vi "FinalBrain.vi"() -> ()   [LabVIEW 2012]
uses:
  <vilib>/imath/engines/lvmath/Plug In/_Char/NIMS_CH_character datatype.ctl
  <vilib>/Utility/inputDevices.llb/closeKeyboard.vi
  <vilib>/Utility/inputDevices.llb/keyboardAcquire.vi
  <vilib>/imath/engines/lvmath2/RunTimeEngine/ErrorHandling/NIMS_Finalize Error.vi
  <vilib>/imath/engines/lvmath2/RunTimeEngine/Managers/WorkSpace/UID Generator.vi
  <vilib>/imath/engines/lvmath2/RunTimeEngine/Managers/SymbolTable/Clear UID.vi
  <vilib>/imath/engines/lvmath2/RunTimeEngine/NodeEndStatement/NIMS_NodeEndStatement_Output.vi
  <instcachedir>/0/NIMS_NodeEndStatement_Output_53EC0D466D134D7ABD903AC30B43404B.lvgen/NIMS_NodeEndStatement_Output_53EC0D466D134D7ABD903AC30B43404B_010.vi
  <instcachedir>/0/NIMS_NodeEndStatement_Output_53EC0D466D134D7ABD903AC30B43404B.lvgen/NIMS_NodeEndStatement_Output_53EC0D466D134D7ABD903AC30B43404B_012.vi
  <vilib>/imath/engines/lvmath2/RunTimeEngine/RunTimeType/NIMS_RunTimeType_From StrictType (excl LVString).vi
  <instcachedir>/0/NIMS_RunTimeType_From StrictType (excl LVString)_AC52D965D0864706932D20A05968E122.lvgen/NIMS_RunTimeType_From StrictType (excl LVString)_AC52D965D0864706932D20A05968E122_000.vi
  <vilib>/imath/engines/lvmath2/RunTimeEngine/LocalVariableDefStatement/MC_LocalVariableDefStatement_Display.vi
  <vilib>/imath/engines/lvmath2/RunTimeEngine/RunTimeType/NIMS_RunTimeType_Set Source Original Bool.vi
  <vilib>/imath/engines/lvmath/Plug In/_Char/NIMS_CH_Character RV to String.vi
  <instcachedir>/0/NIMS_NodeEndStatement_Output_53EC0D466D134D7ABD903AC30B43404B.lvgen/NIMS_NodeEndStatement_Output_53EC0D466D134D7ABD903AC30B43404B_009.vi
  <instcachedir>/0/NIMS_RunTimeType_From StrictType (excl LVString)_AC52D965D0864706932D20A05968E122.lvgen/NIMS_RunTimeType_From StrictType (excl LVString)_AC52D965D0864706932D20A05968E122_001.vi
  <vilib>/imath/engines/lvmath2/RunTimeEngine/Managers/SymbolTable/NIMS_WorkSpace.lvlib
panel:
  out "Fully elapsed":bool
  out "Elapsed Time (s)":dbl
  out "String Received 3":string
  out "BS Timed Out":bool
  out "Base Station":string
  in  "error in (no error)":errorcluster
  in  "Tab Control":T1(tab)
  in  "Read Color":bool
  out "Bump Sensor 2":bool
  out "Distance 2, CM":dbl
  out "IR Volts Nav":dbl
  out "Red":dbl(knob) scale=0.0..50.0
  out "Green":dbl(knob) scale=0.0..50.0
  out "Blue":dbl(knob) scale=0.0..50.0
  out "Color Chosen":u32(colorbox)
  out "Bump Sensor 1":bool
  out "IR Volts Align":dbl
  out "Distance 1, CM":dbl
  in  "stop":bool
  out "Left Arm":i32
  out "Right Arm":i32
  in  "Arm":i32(slide)=1500 scale=500.0..2500.0
  out "Port\nMotor":i32
  out "Starboard\nMotor":i32
  out "Port Speed":i32(knob) scale=1000.0..2000.0
  out "Starboard Speed":i32(knob) scale=1000.0..2000.0
  out "Speed Balance":i32(knob) scale=-600.0..600.0
  in  "Numeric":i32=500
  in  "Arm Override":bool
  in  "Extend":bool
  in  "Initiate Mission":bool
  out "Angle to Target":i32
  out "Distance to Target":i32
  out "Bump 2":bool
  out "Bump  1":bool
  out "Current Target":i32
  out "Obstacle Detected":bool
  out "Primitive Engaged":string
  out "Desired Heading":i32
  out "Target Y":i32
  out "Target X":i32
  out "Current Y":i32
  out "Current X":i32
  out "Current Heading":i32
  out "Target Locations":i32[][](array[numeric])
  out "X Array":dbl[](array[numeric])
  out "Y Array":dbl[](array[numeric])
  in  "Step Size":i32=5
  in  "PC Status":i32=1
  out "String Received":string
  out "return count":u32
  out "bytes written":u32
  out "Blinky":bool
  in  "String":string="$CS1500P1500R1500L1500P1500H   1\n"
  in  "FULLSTOP":bool
  in  "VISA resource name":refnum<visa-resource-name>="COM7"
  # "ROBOT CONTROL VI\nSoftware Phase for Autonomy\n\nVPreston\n4/14/2014"
  # "Thought:\n- Need to calibrate the accelerometer each time, which means that the first step will need to be \nSpinning in place at a set location (likely the landing zone)\n- Is this worth it?  If not, a simple heading can be developed based upon movement from the \ncamera, though this is likely to be glitchy and less reliable....\n\n- Calculate heading with accelerometer in the hindbrain, pass this up to PC\nOR\n- Calculate heading from base station in PC"
  # "Use this tab to make sure your sensors are happy and working properly."
  # "Motor Control"
  # "Direction of thrust"
  # "Purple Target - 80, 230\nYellow Target - \nRed Target - 37, 78 \nGreen Target - 258, 43 \nBlue Target - 492, 63"
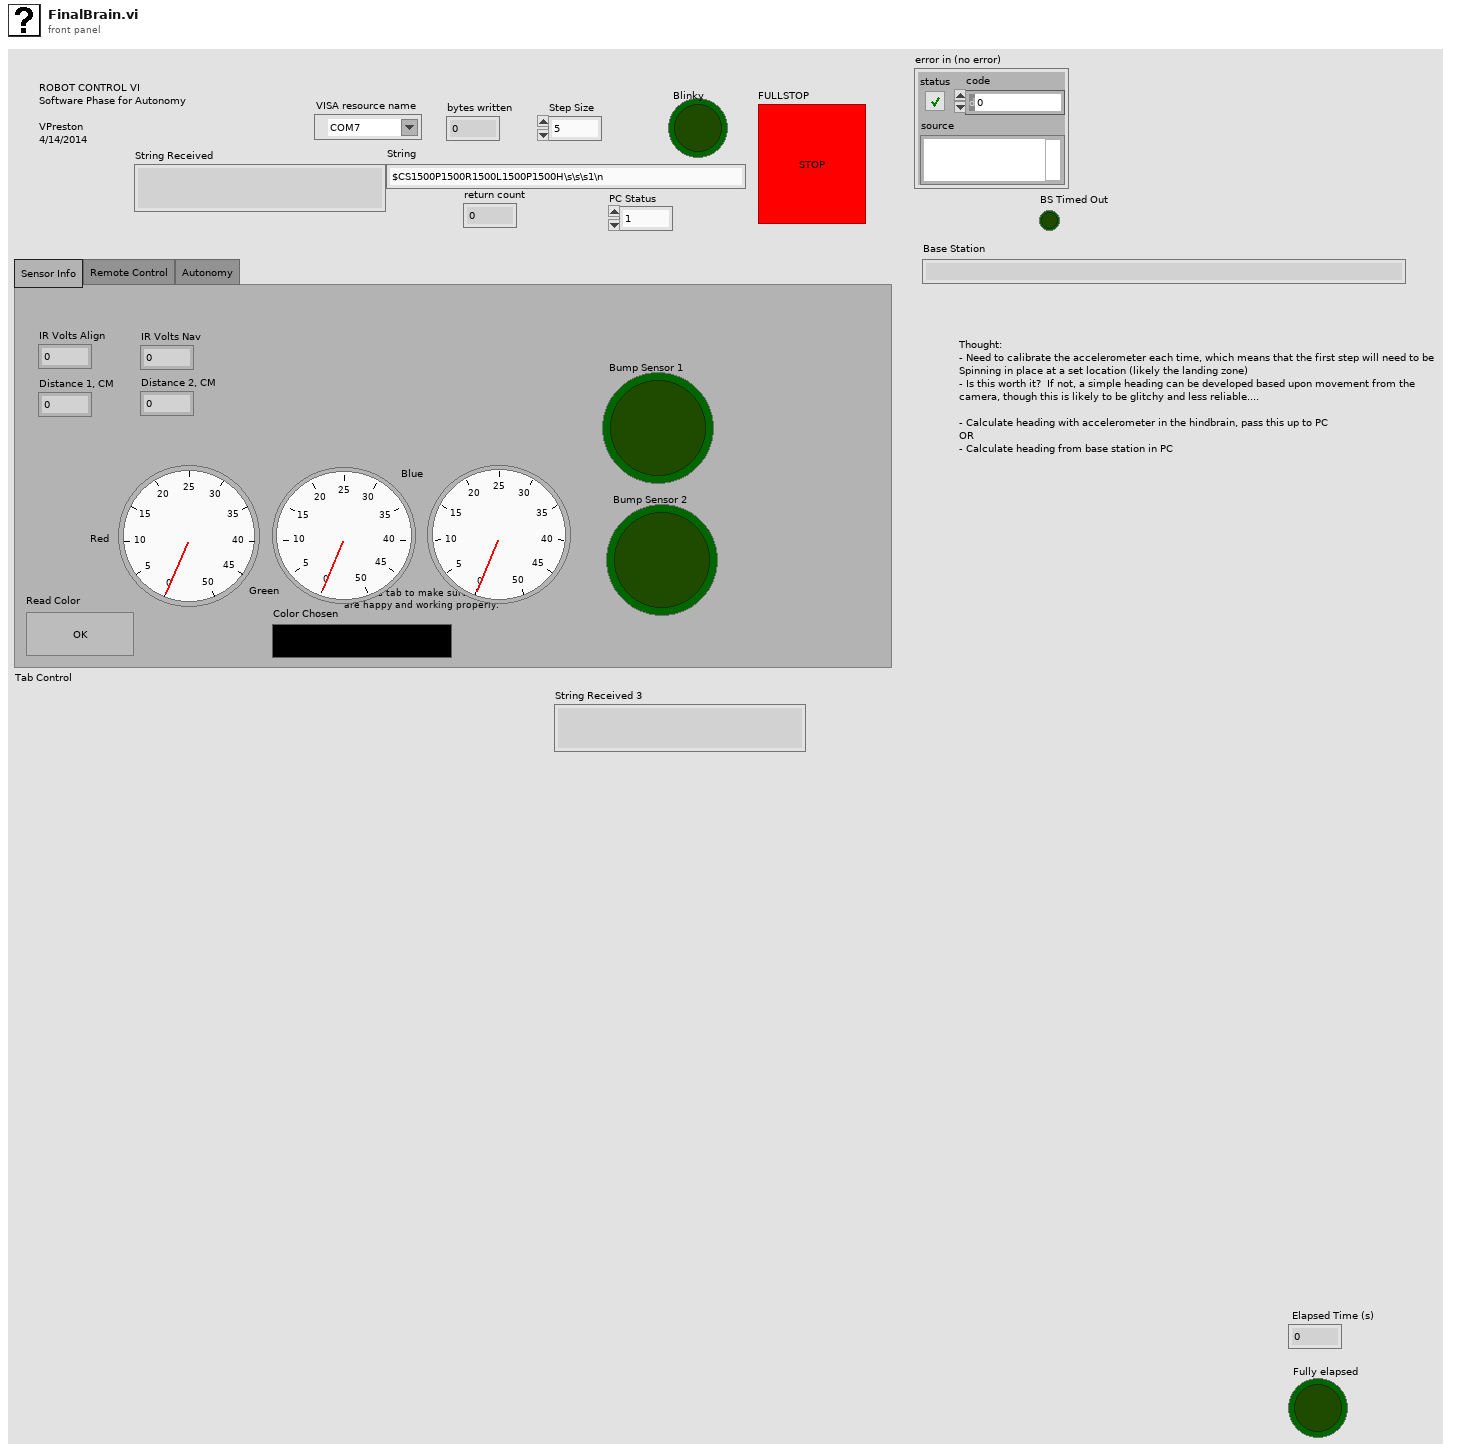
[diagram p1: front panel]
types:
  T1 = enum32{"Sensor Info", "Remote Control", "Autonomy"}
  T2 = enum16{"0", "1", "2", "3", "4", "5", "6", "7", "8", "9", "A", "B", "C", "D", "E", "F", "G", "H", "I", "J", "K", "L", "M", "N", "O", "P", "Q", "R", "S", "T", "U", "V", "W", "X", "Y", "Z", "F1", "F2", "F3", "F4", "F5", "F6", "F7", "F8", "F9", "F10", "F11", "F12", "F13", "F14", "F15", "ADD", "BACK", "BACKSLASH", "CAPITAL", "COMMA", "DECIMAL", "DELETE", "DIVIDE", "DOWN", "END", "EQUALS", "ESCAPE", "GRAVE (`)", "HOME", "INSERT", "LBRACKET", "LCONTROL", "LEFT", "L ALT", "LSHIFT", "LWIN", "MINUS", "MULTIPLY", "NEXT", "NUMLOCK", "NUMPAD_0", "NUMPAD_1", "NUMPAD_2", "NUMPAD_3", "NUMPAD_4", "NUMPAD_5", "NUMPAD_6", "NUMPAD_7", "NUMPAD_8", "NUMPAD_9", "PAUSE", "PERIOD", "PRIOR (PG UP)", "RBRACKET", "RCONTROL", "RETURN", "RIGHT", "R ALT", "RSHIFT", "RWIN", "SCROLL", "SEMICOLON", "SLASH", "SPACE", "SUBTRACT", "TAB", "UP", "ENTER (num pad)", "' (quote)"}[]
  T3 = enum16{"0", "1", "2", "3", "4", "5", "6", "7", "8", "9", "A", "B", "C", "D", "E", "F", "G", "H", "I", "J", "K", "L", "M", "N", "O", "P", "Q", "R", "S", "T", "U", "V", "W", "X", "Y", "Z", "F1", "F2", "F3", "F4", "F5", "F6", "F7", "F8", "F9", "F10", "F11", "F12", "F13", "F14", "F15", "ADD", "BACK", "BACKSLASH", "CAPITAL", "COMMA", "DECIMAL", "DELETE", "DIVIDE", "DOWN", "END", "EQUALS", "ESCAPE", "GRAVE (`)", "HOME", "INSERT", "LBRACKET", "LCONTROL", "LEFT", "L ALT", "LSHIFT", "LWIN", "MINUS", "MULTIPLY", "NEXT", "NUMLOCK", "NUMPAD_0", "NUMPAD_1", "NUMPAD_2", "NUMPAD_3", "NUMPAD_4", "NUMPAD_5", "NUMPAD_6", "NUMPAD_7", "NUMPAD_8", "NUMPAD_9", "PAUSE", "PERIOD", "PRIOR (PG UP)", "RBRACKET", "RCONTROL", "RETURN", "RIGHT", "R ALT", "RSHIFT", "RWIN", "SCROLL", "SEMICOLON", "SLASH", "SPACE", "SUBTRACT", "TAB", "UP", "ENTER (num pad)", "' (quote)"}
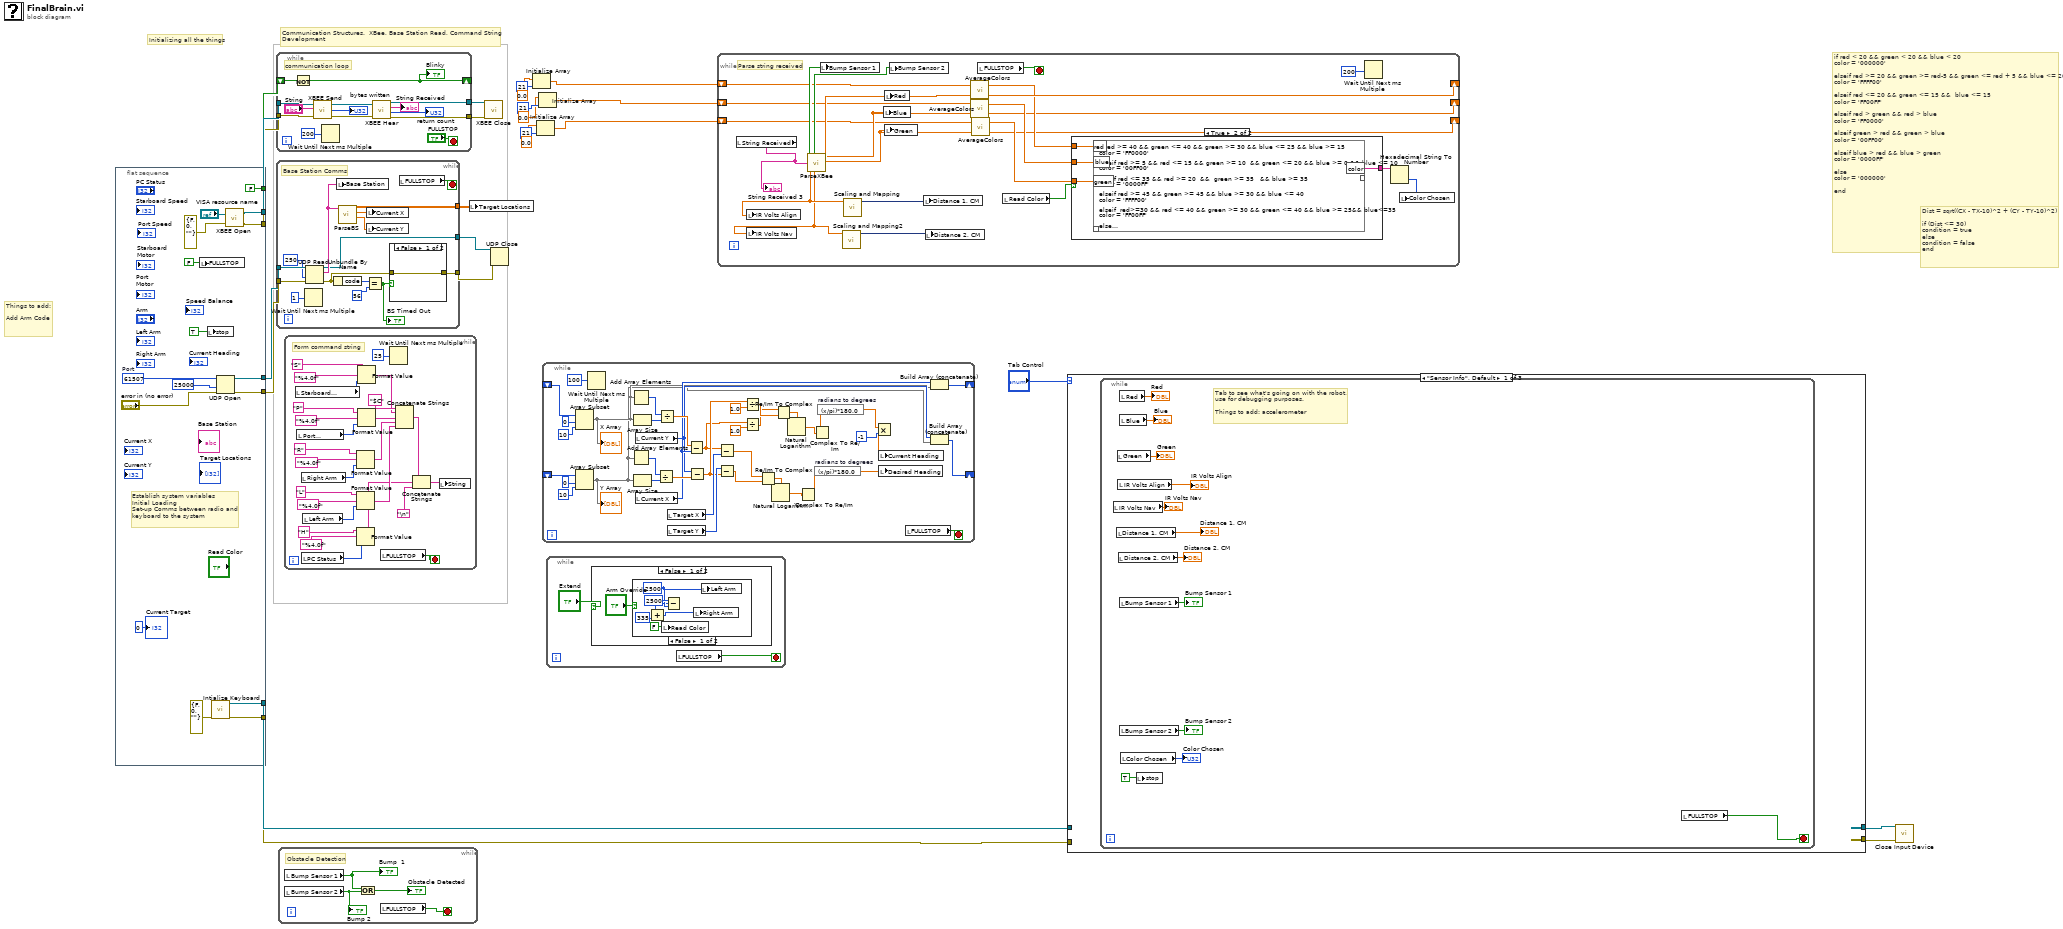
[diagram p0: block diagram]
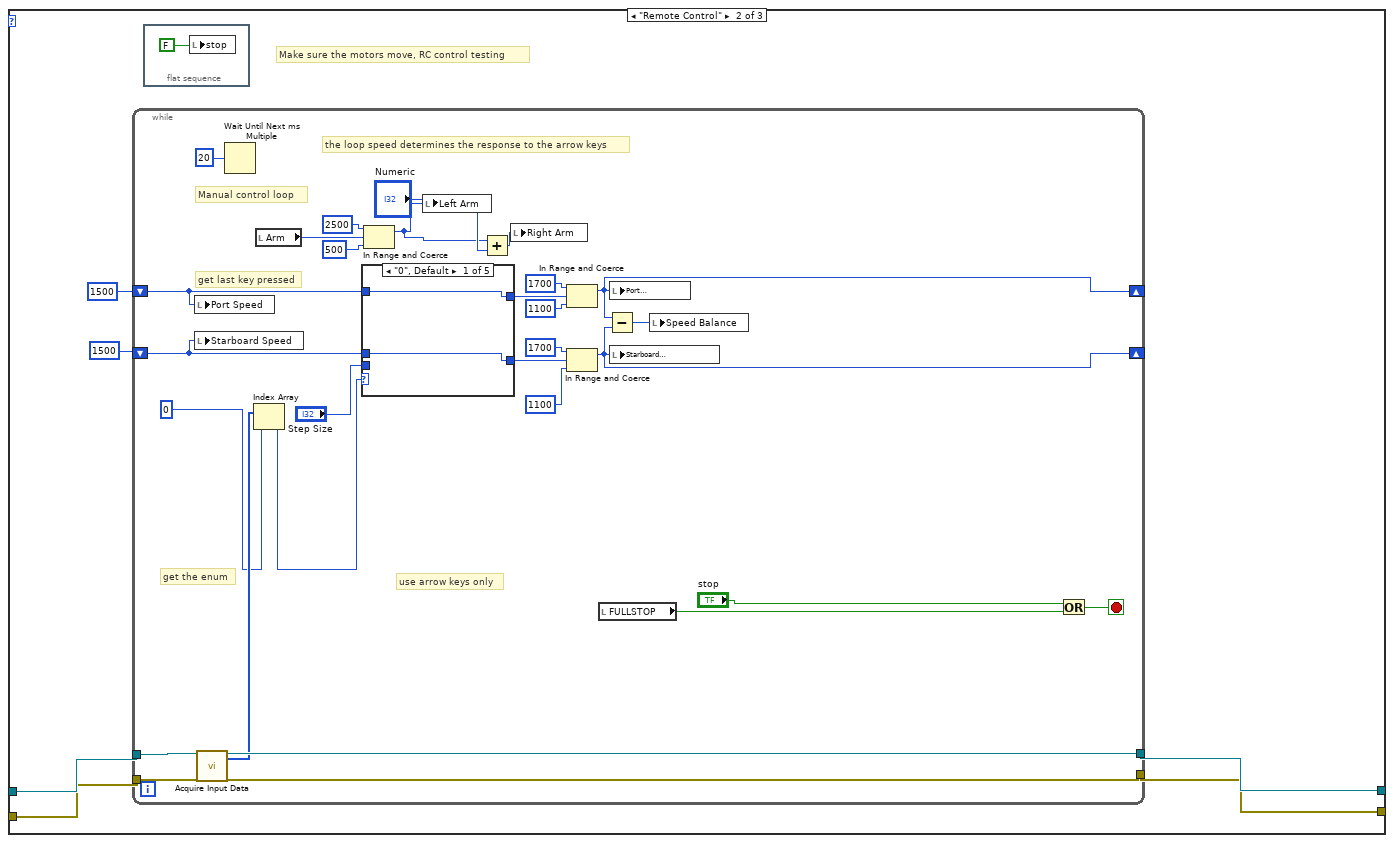
[diagram p2: hidden frame]
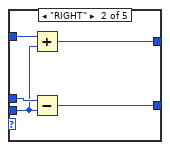
[diagram p3: hidden frame]
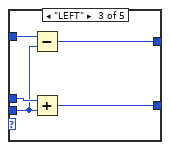
[diagram p4: hidden frame]
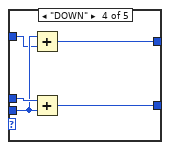
[diagram p5: hidden frame]
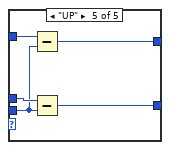
[diagram p6: hidden frame]
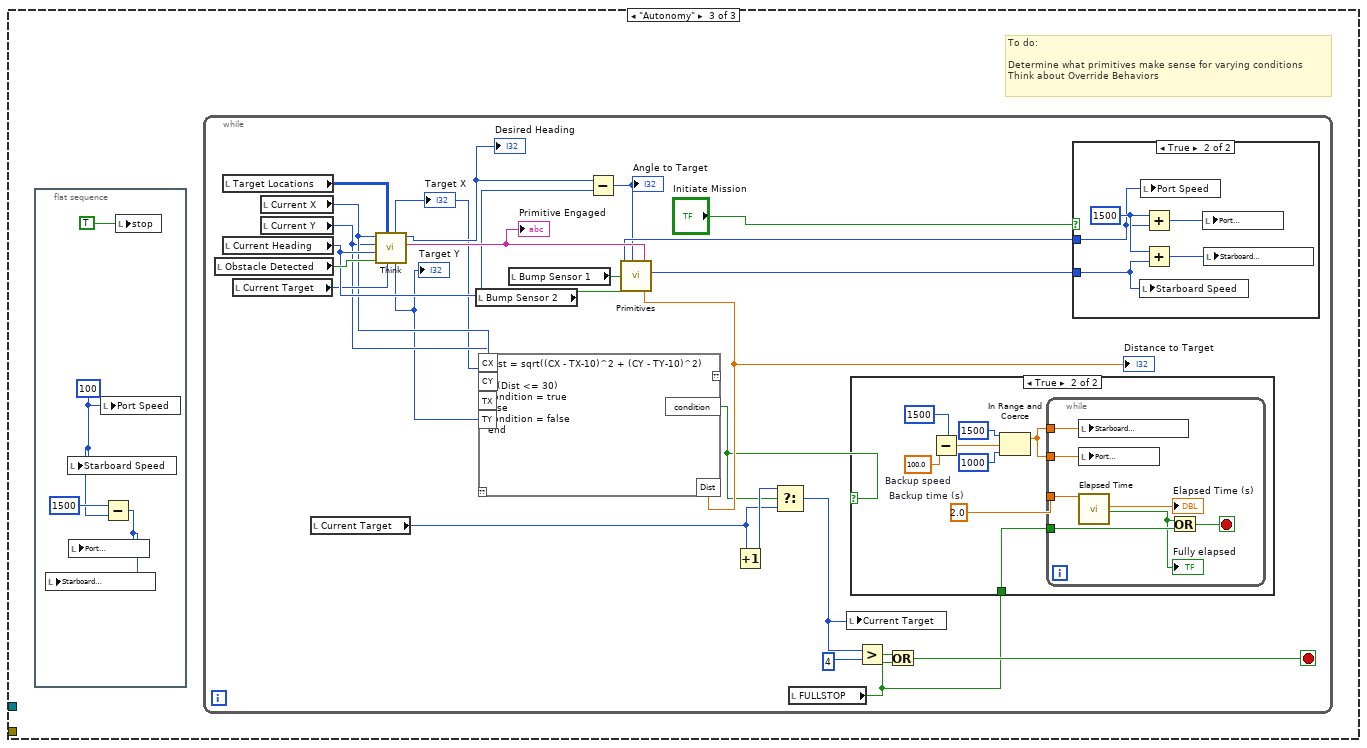
[diagram p7: hidden frame]
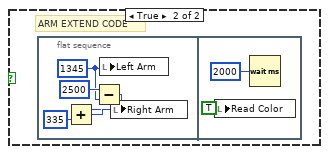
[diagram p11: hidden frame]
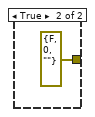
[diagram p12: hidden frame]
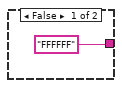
[diagram p13: hidden frame]
diagram:
  # "Dist = sqrt((CX - TX-10)^2 + (CY - TY-10)^2)\n\nif (Dist <= 30)\ncondition = true\nelse\ncondition = false\nend"
  # "if red < 20 && green < 20 && blue < 20\ncolor = '000000'\n\nelseif red >= 20 && green >= red-5 && green <= red + 5 && blue <= 20\ncolor = 'FFFF00'\n\nelseif red <= 20 && green <= 15 &&  blue <= 15\ncolor = 'FF00FF'\n\nelseif red > green && red > blue\ncolor = 'FF0000'\n\nelseif green > red && green > blue\ncolor = '00FF00'\n\nelseif blue > red && blue > green\ncolor = '0000FF' \n\nelse\ncolor = '000000'\n\nend"
  # "Initializing all the things"
  # "Communication Structures.  XBee, Base Station Read, Command String Development"
  # "Things to add: \n\nAdd Arm Code"
  n1 = flat-sequence {
    tunnel: [w40] -> w24
    tunnel: [w28] -> w23
    tunnel: [FALSE] -> w20
    tunnel: [w35] -> w19
    tunnel: [w34] -> w18
    tunnel: [w27] -> w12
    tunnel: [w29] -> w15
    frame #0 {
      w31 = u16 61507  # Port
      # "Establish system variables\nInitial Loading\nSet-up Comms between radio and\nkeyboard to the system"
      n2 = local write "FULLSTOP"(FALSE) -> ()
      n3 = local write "stop"(TRUE) -> ()
      n4 = call <vilib>:"Intialize Keyboard.vi"("error in (no error)"=errorcluster {"status"=FALSE, "code"=0, "source"=""}) -> ("error out"=w34:errorcluster, "device ID"=w35:refnum<k1>)  [unwired: 9 in]
      n5 = UDP Open(8:"error in (no error)", 9:25000 ("timeout ms (25000)"), 11:w31) -> (port=w27:refnum<k16>, 0:w29:errorcluster)  [unwired: 2 in, 1 out]
      n6 = call "XBEE Open.vi"("error in"=errorcluster {"status"=FALSE, "code"=0, "source"=""}, "VISA resource name"="VISA resource name") -> ("error out"=w28:errorcluster, "VISA resource name out"=w40:refnum<visa-resource-name>)
      "Current Target" <- 0
    }
  }
  n7 = while {
    tunnel: w24 -> [w53]
    tunnel: w23 -> [w52]
    tunnel: [w47] -> w22
    tunnel: [w46] -> w21
    shift-right: [w50] -> _
    shift-left: w20 -> [w51]
    stop <- "FULLSTOP" stop-if-true
    # "communication loop"
    n8 = Not(x=w51) -> (.not. x?=w50:bool)
    "Blinky" <- w50
    n9 = call "XBEE Send.vi"("error in (no error)"=w52, "String"="String", "VISA resource name"=w53) -> ("error out"=w43:errorcluster, "return count"=→"bytes written":u32, "VISA resource name out"=w44:refnum<visa-resource-name>)
    n10 = Wait Until Next ms Multiple(millisecond multiple=u32 200) -> ()  [unwired: 1 out]
    n11 = call "XBEE Hear.vi"("VISA resource name"=w44, "error in (no error)"=w43) -> ("VISA resource name out"=w47:refnum<visa-resource-name>, "String Received"=→"String Received":string, "return count"=→"return count":u32, "error out"=w46:errorcluster)
  }
  n12 = while {
    tunnel: w12 -> [w69]
    tunnel: w15 -> [w68]
    tunnel: [w57] -> w14
    tunnel: [w56] -> w13
    tunnel: [w55] -> w1
    stop <- w61 stop-if-true
    # "Base Station Comms"
    n13 = Wait Until Next ms Multiple(millisecond multiple=u32 1) -> ()  [unwired: 1 out]
    n14 = UDP Read(connection ID=w69, timeout ms (25000)=250, 8:w68) -> (data out=w60:string, error out=w64:errorcluster, 3:w57:refnum<k16>)  [unwired: 1 in, 2 out]
    n15 = Unbundle By Name(w64) -> ("code"=w63:i32)
    n16 = local write "Base Station"(w60) -> ()
    n17 = call "ParseBS.vi"("BS String"=w60) -> ("Y Pos"=w58:dbl, "X Pos"=w59:dbl, "Targets!"=w55:dbl[][])  [unwired: 7 in]
    n18 = Equal?(x=w63, y=56) -> (x = y?=w62:bool)
    "BS Timed Out" <- w62
    n19 = local write "Current X"(w59) -> ()
    n20 = local write "Current Y"(w58) -> ()
    n21 = case shown="False" w62 {
      tunnel: [w70 errorcluster {"status"=FALSE, "code"=0, "source"=""} ("error out")] -> w56
      tunnel: w64 -> [w70 _]
      frame False {
      }
      frame True {
      }
    }
    n22 = local read "FULLSTOP"() -> (w61:bool)
  }
  n23 = while {
    stop <- w75 stop-if-true
    # "Obstacle Detection"
    n24 = local read "Bump Sensor 1"() -> (w74:bool)
    "Bump  1" <- w74
    n25 = local read "Bump Sensor 2"() -> (w73:bool)
    "Bump 2" <- w73
    n26 = Or(x=w74, y=w73) -> (x .or. y?=→"Obstacle Detected":bool)
    n27 = local read "FULLSTOP"() -> (w75:bool)
  }
  n28 = while {
    stop <- w101 stop-if-true
    # "Form command string"
    n29 = local read "Starboard\nMotor"() -> (w98:i32)
    n30 = local read "Port\nMotor"() -> (w95:i32)
    n31 = local read "Right Arm"() -> (w89:i32)
    n32 = local read "PC Status"() -> (w80:i32)
    n33 = local read "Left Arm"() -> (w86:i32)
    n34 = Format Value(string ("")="R", format string="%4.0f", value (0)=w89) -> (output string=w85:string)
    n35 = Format Value(string ("")="H", format string="%4.0f", value (0)=w80) -> (output string=w77:string)
    n36 = Format Value(string ("")="L", format string="%4.0f", value (0)=w86) -> (output string=w84:string)
    n37 = Format Value(string ("")="S", format string="%4.0f", value (0)=w98) -> (output string=w93:string)
    n38 = Format Value(string ("")="P", format string="%4.0f", value (0)=w95) -> (output string=w92:string)
    n39 = local read "FULLSTOP"() -> (w101:bool)
    n40 = Wait Until Next ms Multiple(millisecond multiple=u32 25) -> ()  [unwired: 1 out]
    n41 = Concatenate Strings("$C", w93, w92, w85, w84) -> (w79:string)
    n42 = Concatenate Strings(w79, w77, "\n") -> (w83:string)
    n43 = local write "String"(w83) -> ()
  }
  n44 = local write "Target Locations"(w1) -> ()
  n45 = call "XBEE Close.vi"("error in (no error)"=w21, "VISA resource name"=w22) -> ()
  n46 = UDP Close(connection ID=w14, 8:w13) -> ()  [unwired: 2 out]
  n47 = Initialize Array(0.0 ("element"), 21 ("dimension size")) -> (w11:dbl[])
  n48 = Initialize Array(0.0 ("element"), 21 ("dimension size")) -> (w3:dbl[])
  n49 = Initialize Array(0.0 ("element"), 21 ("dimension size")) -> (w4:dbl[])
  n50 = while {
    shift-right: [w121] -> _
    shift-left: _ -> [w141]
    shift-right: [w118] -> _
    shift-left: _ -> [w135]
    stop <- w134 stop-if-true
    n51 = Array Subset(array=w141, index=0, length=10) -> (w117:i32[])
    "X Array" <- w117
    n52 = Array Subset(array=w135, index=0, length=10) -> (w116:i32[])
    "Y Array" <- w116
    n53 = Wait Until Next ms Multiple(millisecond multiple=100) -> ()  [unwired: 1 out]
    n54 = Add Array Elements(numeric array=w117) -> (sum=w132:i32)
    n55 = Add Array Elements(numeric array=w116) -> (sum=w130:i32)
    n56 = Array Size(array=w117) -> (size(s)=w131:i32)
    n57 = Array Size(array=w116) -> (size(s)=w129:i32)
    n58 = local read "Current Y"() -> (w119:i32)
    n59 = local read "Current X"() -> (w120:i32)
    n60 = Divide(x=w130, y=w129) -> (x/y=w124:dbl)
    n61 = Divide(x=w132, y=w131) -> (x/y=w122:dbl)
    n62 = local read "Target X"() -> (w126:i32)
    n63 = local read "Target Y"() -> (w125:i32)
    n64 = Subtract(x=w122, y=w120) -> (x-y=w115:dbl)
    n65 = Subtract(x=w119, y=w124) -> (x-y=w123:dbl)
    n66 = Subtract(x=w115, y=w126) -> (x-y=w104:dbl)
    n67 = Subtract(x=w125, y=w123) -> (x-y=w105:dbl)
    n68 = Divide(x=w123, y=1.0) -> (x/y=w111:dbl)
    n69 = Divide(x=w115, y=1.0) -> (x/y=w110:dbl)
    n70 = Re/Im To Complex(1:w105, 2:w104) -> (0:w106:cdb)
    n71 = Natural Logarithm(1:w106) -> (0:w103:cdb)
    n72 = Re/Im To Complex(1:w111, 2:w110) -> (0:w109:cdb)
    n73 = Natural Logarithm(1:w109) -> (0:w108:cdb)
    n74 = Complex To Re/Im(x + iy=w103) -> (y=w102:dbl)  [unwired: 1 out]
    n75 = Complex To Re/Im(x + iy=w108) -> (y=w107:dbl)  [unwired: 1 out]
    n76 = expression code="(x/pi)*180.0" "radians to degrees"(w102) -> (w133:dbl)
    n77 = expression code="(x/pi)*180.0" "radians to degrees"(w107) -> (w113:dbl)
    n78 = Multiply(x=w113, y=-1) -> (x*y=w112:dbl)
    n79 = local write "Current Heading"(w112) -> ()
    n80 = local write "Desired Heading"(w133) -> ()
    n81 = local read "FULLSTOP"() -> (w134:bool)
    n82 = Build Array (concatenate)(w120, w117) -> (w121:i32[])
    n83 = Build Array (concatenate)(w119, w116) -> (w118:i32[])
  }
  n84 = while {
    stop <- w143 stop-if-true
    n85 = case shown="False" "Extend" {
      frame False {
        n86 = case shown="False" "Arm Override" {
          frame False {
            w148 = 2500 ("Left Arm")
            n87 = local write "Read Color"(FALSE ("Read Color")) -> ()
            n88 = Subtract(x=2500, y=w148) -> (x-y=w147:i32)
            n89 = Add(x=w147, y=335) -> (x+y=w146:i32)
            n90 = local write "Right Arm"(w146) -> ()
            n91 = local write "Left Arm"(w148) -> ()
          }
          frame True {
          }
        }
      }
      frame True {
        # "ARM EXTEND CODE"
        n92 = flat-sequence {
          frame #0 {
            w152 = 1345 ("Left Arm")
            n93 = Subtract(x=2500, y=w152) -> (x-y=w153:i32)
            n94 = Add(x=w153, y=335) -> (x+y=w154:i32)
            n95 = local write "Left Arm"(w152) -> ()
            n96 = local write "Right Arm"(w154) -> ()
          }
          frame #1 {
            n97 = local write "Read Color"(TRUE ("Read Color")) -> ()
            n98 = Wait (ms)(milliseconds to wait=u32 2000) -> ()  [unwired: 1 out]
          }
        }
      }
    }
    n99 = local read "FULLSTOP"() -> (w143:bool)
  }
  n100 = while {
    shift-right: [w171] -> _
    shift-left: w11 -> [w172]
    shift-right: [w163] -> _
    shift-left: w4 -> [w164]
    shift-right: [w161] -> _
    shift-left: w3 -> [w162]
    stop <- w165 stop-if-true
    # "Parse string received"
    n101 = local read "String Received"() -> (w159:string)
    "String Received 3" <- w159
    n102 = call "ParseXBee.vi"("XBee String"=w159) -> ("Bump 1"=w177:bool, "Bump 2"=w176:bool, "IR Align"=w175:dbl, "IR Nav"=w174:dbl, "Red"=w173:dbl, "Blue"=w169:dbl, "Green"=w167:dbl)  [unwired: 3 in]
    n103 = local write "IR Volts Align"(w175) -> ()
    n104 = local write "IR Volts Nav"(w174) -> ()
    n105 = local write "Bump Sensor 1"(w177) -> ()
    n106 = call "Scaling and Mapping2"("Signals"=w174) -> ("Scaled Signals"=w178:dynamicdata)  [unwired: 9 in, 1 out]
    n107 = call "Scaling and Mapping"("Signals"=w175) -> ("Scaled Signals"=w179:dynamicdata)  [unwired: 9 in, 1 out]
    n108 = local write "Blue"(w169) -> ()
    n109 = local write "Red"(w173) -> ()
    n110 = local write "Green"(w167) -> ()
    n111 = local write "Bump Sensor 2"(w176) -> ()
    n112 = local write "Distance 1, CM"(w179) -> ()
    n113 = local write "Distance 2, CM"(w178) -> ()
    n114 = call "AverageColors.vi"("ColorData"=w173, "CurrentArray"=w172) -> ("UpdatedArray"=w171:dbl[], "Average"=w170:dbl)
    n115 = call "AverageColors.vi"("ColorData"=w169, "CurrentArray"=w164) -> ("UpdatedArray"=w163:dbl[], "Average"=w168:dbl)
    n116 = call "AverageColors.vi"("ColorData"=w167, "CurrentArray"=w162) -> ("UpdatedArray"=w161:dbl[], "Average"=w166:dbl)
    n117 = local read "FULLSTOP"() -> (w165:bool)
    n118 = local read "Read Color"() -> (w160:bool)
    n119 = case shown="True" w160 {
      tunnel: ["FFFFFF" w186] -> w181
      tunnel: w170 -> [_ w185]
      tunnel: w168 -> [_ w184]
      tunnel: w166 -> [_ w183]
      frame False {
      }
      frame True {
        n120 = mathscript code="if red >= 40 && green <= 40 && green >= 30 && blue <= 25 && blue >= 15\ncolor = 'FF0000'\n\nelseif red >= 5 && red <= 15 && green >= 10  && green <= 20 && blue >= 0 && blue <= 10\ncolor = '00FF00'\n\nelseif red <= 35 && red >= 20  &&  green >= 35   && blue >= 35 \ncolor = '0000FF'\n\nelseif red >= 45 && green >= 45 && blue >= 30 && blue <= 40\ncolor = 'FFFF00'\n\nelseif  red>=30 && red <= 40 && green >= 30 && green <= 40 && blue >= 25&& blue<=35\ncolor = 'FF00FF'\n\nelse\ncolor = '000000'\n\nend"("red"=w185, "blue"=w184, "green"=w183) -> ("color"=w186:string)  [unwired: 1 in, 1 out]
      }
    }
    n121 = Wait Until Next ms Multiple(millisecond multiple=200) -> ()  [unwired: 1 out]
    n122 = Hexadecimal String To Number(string=w181) -> (number=w180:u32)  [unwired: 2 in, 1 out]
    n123 = local write "Color Chosen"(w180) -> ()
  }
  n124 = case shown="\"Sensor Info\", Default" "Tab Control" {
    tunnel: w19 -> [_ w540 _]
    tunnel: w18 -> [_ w539 _]
    tunnel: [_ w536 _] -> w17
    tunnel: [_ w535 _] -> w16
    frame "Sensor Info", Default {
      n125 = while {
        stop <- w523 stop-if-true
        # "Tab to see what's going on with the robot, \nuse for debugging purposes.  \n\nThings to add: accelerometer"
        n126 = local read "IR Volts Nav"() -> (→"IR Volts Nav":dbl)
        n127 = local read "Distance 1, CM"() -> (→"Distance 1, CM":dbl)
        n128 = local read "Green"() -> (→"Green":dbl)
        n129 = local read "IR Volts Align"() -> (→"IR Volts Align":dbl)
        n130 = local read "Distance 2, CM"() -> (→"Distance 2, CM":dbl)
        n131 = local read "Bump Sensor 1"() -> (→"Bump Sensor 1":bool)
        n132 = local read "Bump Sensor 2"() -> (→"Bump Sensor 2":bool)
        n133 = local read "Red"() -> (→"Red":dbl)
        n134 = local read "Blue"() -> (→"Blue":dbl)
        n135 = local read "Color Chosen"() -> (→"Color Chosen":u32)
        n136 = local write "stop"(TRUE) -> ()
        n137 = local read "FULLSTOP"() -> (w523:bool)
      }
    }
    frame "Remote Control" {
      # "Make sure the motors move, RC control testing"
      n138 = while {
        tunnel: [w570] -> w535
        tunnel: [w569] -> w536
        shift-right: [w553] -> _
        shift-left: 1500 -> [w555]
        shift-right: [w552] -> _
        shift-left: 1500 -> [w554]
        tunnel: w540 -> [w546]
        tunnel: w539 -> [w545]
        stop <- w547 stop-if-true
        # "use arrow keys only"
        # "Manual control loop"
        # "get the enum"
        # "the loop speed determines the response to the arrow keys"
        # "get last key pressed"
        n139 = local write "Port Speed"(w554) -> ()
        n140 = local write "Starboard Speed"(w555) -> ()
        n141 = call-poly <vilib>:"Acquire Input Data.vi"("device ID"=w546, "error in (no error)"=w545) -> ("device ID"=w569:refnum<k1>, "keys pressed"=w568:T2, "error out"=w570:errorcluster)  [unwired: 15 in]
        n142 = Wait Until Next ms Multiple(millisecond multiple=u32 20) -> ()  [unwired: 1 out]
        n143 = Index Array(array=w568, index=0) -> (element=w566:T3)
        n144 = local read "Arm"() -> (w550:i32)
        n145 = case shown="\"0\", Default" w566 {
          tunnel: w555 -> [w572 w574 w579 w587 w592]
          tunnel: [w572 w575 w580 w586 w591] -> w564
          tunnel: w554 -> [w571 w577 w581 w584 w590]
          tunnel: [w571 w576 w582 w583 w588] -> w556
          tunnel: "Step Size" -> [_ w573 w578 w585 w589]
          frame "0", Default {
          }
          frame "RIGHT" {
            n146 = Add(x=w577, y=w573) -> (x+y=w576:i32)
            n147 = Subtract(x=w574, y=w573) -> (x-y=w575:i32)
          }
          frame "LEFT" {
            n148 = Subtract(x=w581, y=w578) -> (x-y=w582:i32)
            n149 = Add(x=w579, y=w578) -> (x+y=w580:i32)
          }
          frame "DOWN" {
            n150 = Add(x=w585, y=w584) -> (x+y=w583:i32)
            n151 = Add(x=w587, y=w585) -> (x+y=w586:i32)
          }
          frame "UP" {
            n152 = Subtract(x=w590, y=w589) -> (x-y=w588:i32)
            n153 = Subtract(x=w592, y=w589) -> (x-y=w591:i32)
          }
        }
        n154 = In Range and Coerce(upper limit=2500, x=w550, lower limit=500) -> (coerced(x)=w542:i32)  [unwired: 1 out]
        n155 = local write "Left Arm"(w542) -> ()
        n156 = Add(x=w542, y="Numeric") -> (x+y=w543:i32)
        n157 = local write "Right Arm"(w543) -> ()
        n158 = In Range and Coerce(upper limit=1700, x=w556, lower limit=1100) -> (coerced(x)=w552:i32)  [unwired: 1 out]
        n159 = In Range and Coerce(upper limit=1700, x=w564, lower limit=1100) -> (coerced(x)=w553:i32)  [unwired: 1 out]
        n160 = local read "FULLSTOP"() -> (w548:bool)
        n161 = Subtract(x=w552, y=w553) -> (x-y=w551:i32)
        n162 = local write "Port\nMotor"(w552) -> ()
        n163 = local write "Starboard\nMotor"(w553) -> ()
        n164 = local write "Speed Balance"(w551) -> ()
        n165 = Or(x="stop", y=w548) -> (x .or. y?=w547:bool)
      }
      n166 = flat-sequence {
        frame #0 {
          n167 = local write "stop"(FALSE) -> ()
        }
      }
    }
    frame "Autonomy" {
      # "To do:\n\nDetermine what primitives make sense for varying conditions\nThink about Override Behaviors"
      n168 = flat-sequence {
        frame #0 {
          w739 = 100
          n169 = local write "Starboard Speed"(w739) -> ()
          n170 = local write "Port Speed"(w739) -> ()
          n171 = Subtract(x=1500, y=w739) -> (x-y=w738:i32)
          n172 = local write "Starboard\nMotor"(w738) -> ()
          n173 = local write "Port\nMotor"(w738) -> ()
          n174 = local write "stop"(TRUE) -> ()
        }
      }
      n175 = while {
        stop <- w601 stop-if-true
        n176 = local read "Obstacle Detected"() -> (w616:bool)
        n177 = local read "Target Locations"() -> (w617:i32[][])
        n178 = local read "Current Heading"() -> (w611:i32)
        n179 = local read "Current Target"() -> (w608:i32)
        n180 = local read "Current X"() -> (w606:i32)
        n181 = local read "Current Y"() -> (w605:i32)
        n182 = local read "Current Target"() -> (w597:i32)
        n183 = call "Think.vi"("Target"=w608, "Target Locations"=w617, "Override Engaged"=w616, "Current Heading"=w611, "Y Position"=w605, "X Position"=w606) -> ("Executable Primitive"=w615:string, "Desired Heading"=w612:i32, "Desired Y"=w603:i32, "Desired X"=w604:i32)  [unwired: 2 in]
        "Target Y" <- w603
        "Desired Heading" <- w612
        "Primitive Engaged" <- w615
        "Target X" <- w604
        n184 = local read "Bump Sensor 2"() -> (w613:bool)
        n185 = mathscript code="Dist = sqrt((CX - TX-10)^2 + (CY - TY-10)^2)\n\nif (Dist <= 30)\ncondition = true\nelse\ncondition = false\nend"("CX"=w606, "CY"=w605, "TX"=w604, "TY"=w603) -> ("Dist"=w599:cdb, "condition"=w593:bool)  [unwired: 1 in, 1 out]
        "Distance to Target" <- w599
        n186 = local read "Bump Sensor 1"() -> (w614:bool)
        n187 = Subtract(x=w612, y=w611) -> (x-y=w600:i32)
        "Angle to Target" <- w600
        n188 = call "Primitives.vi"("Angle to Target"=w600, "Bump 1"=w614, "Bump 2"=w613, "Primitive"=w615, "Distance to Target"=w599) -> ("Port Speed"=w609:i32, "Starboard Speed"=w610:i32)  [unwired: 2 in]
        n189 = Increment(x=w597) -> (x+1=w598:i32)
        n190 = Select(t=w598, s=w593, f=w597) -> (s? t:f=w596:i32)
        n191 = local read "FULLSTOP"() -> (w594:bool)
        n192 = local write "Current Target"(w596) -> ()
        n193 = case shown="True" w593 {
          tunnel: w594 -> [_ w618]
          frame False {
          }
          frame True {
            w621 = 100.0  # Backup speed
            w625 = 2.0  # Backup time (s)
            n194 = Subtract(x=1500, y=w621) -> (x-y=w619:dbl)
            n195 = In Range and Coerce(upper limit=1500, x=w619, lower limit=1000) -> (coerced(x)=w622:dbl)  [unwired: 1 out]
            n196 = while {
              tunnel: w625 -> [w632]
              tunnel: w622 -> [w630]
              tunnel: w622 -> [w629]
              tunnel: w618 -> [w628]
              stop <- w626 stop-if-true
              n197 = local write "Starboard\nMotor"(w630) -> ()
              n198 = local write "Port\nMotor"(w629) -> ()
              n199 = call "Elapsed Time"("Time Target (s)"=w632) -> ("Elapsed Time (s)"=→"Elapsed Time (s)":dbl, "Time has Elapsed"=w627:bool)  [unwired: 11 in, 6 out]
              "Fully elapsed" <- w627
              n200 = Or(x=w627, y=w628) -> (x .or. y?=w626:bool)
            }
          }
        }
        n201 = Greater?(x=w596, y=4) -> (0:w602:bool)
        n202 = Or(x=w602, y=w594) -> (x .or. y?=w601:bool)
        n203 = case shown="True" "Initiate Mission" {
          tunnel: w610 -> [_ w637]
          tunnel: w609 -> [_ w634]
          frame False {
          }
          frame True {
            w635 = 1500
            n204 = local write "Starboard Speed"(w637) -> ()
            n205 = local write "Port Speed"(w634) -> ()
            n206 = Add(x=w635, y=w634) -> (x+y=w633:i32)
            n207 = Add(x=w635, y=w637) -> (x+y=w636:i32)
            n208 = local write "Port\nMotor"(w633) -> ()
            n209 = local write "Starboard\nMotor"(w636) -> ()
          }
        }
      }
    }
  }
  n210 = call-poly <vilib>:"Close Input Device.vi"("error in (no error)"=w16, "device ID"=w17) -> ()  [unwired: 8 in, 1 out]
